vi "Do.vi"(8 "error in (no error)":errorcluster, 10 "Actor in":refnum<class "Actor.lvclass">, 11 "PID Actor Msg":refnum<class "PID Actor Msg.lvclass">) -> (0 "error out":errorcluster, 2 "Actor out":refnum<class "Actor.lvclass">)   [LabVIEW 2024, in "PID Actor.lvlib" / "PID Actor Msg.lvclass"]
doc: "(<B>Filename</B>: Actor Framework.lvlib:Message.lvclass:Do.vi)\n\nDefines what a message does when it is received by an actor. Generally, a message instructs an actor to invoke one of its methods. By default, this method does nothing. A child class must override it to define behavior. Create a child class by using the Actor Framework Message Maker dialog box."
uses:
  PID Actor Msg.lvclass
  <vilib>/ActorFramework/Actor/Actor.lvclass
  Actor/PID.lvclass
  C:/Program Files (x86)/National Instruments/LabVIEW 2024/vi.lib/ActorFramework/Actor/Actor.lvclass
  PID Actor Msg.lvclass/PID Actor Msg.ctl
  <vilib>/ActorFramework/Message/Message.lvclass
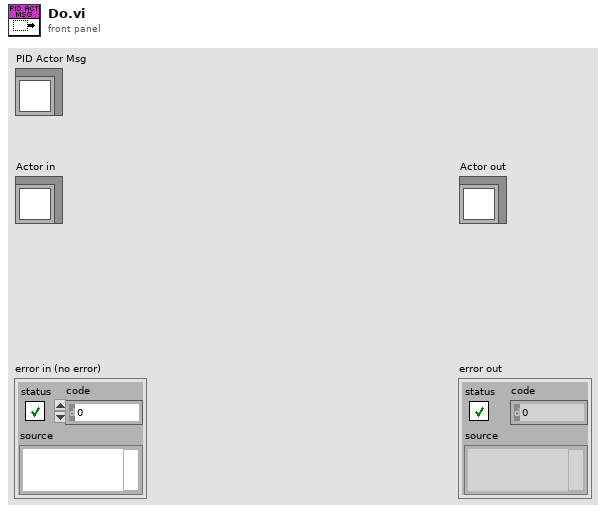
[diagram p1: front panel]
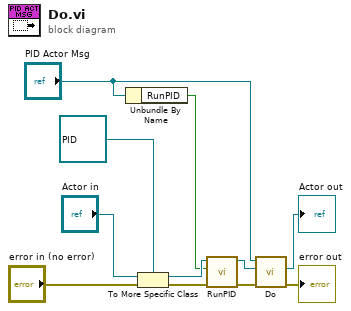
[diagram p0: block diagram]
diagram:
  n1 = Unbundle By Name("PID Actor Msg") -> ("RunPID"=w4:bool)
  n2 = To More Specific Class(target class=refnum<class "PID.lvclass"> refnum ("PID Actor.lvlib:PID.lvclass"), reference="Actor in", error in="error in (no error)") -> (specific class reference=w6:refnum<class "PID.lvclass">, error out=w5:errorcluster)
  n3 = call "RunPID.vi"("error in (no error)"=w5, "Run"=w4, "PID in"=w6) -> ("error out"=w1:errorcluster, "PID out"=w2:refnum<class "PID.lvclass">)  [unwired: 7 in]
  n4 = call-parent "Do.vi"("error in (no error)"=w1, "Actor in"=w2, "Message"="PID Actor Msg") -> ("error out"=→"error out":errorcluster, "Actor out"=→"Actor out":refnum<class "Actor.lvclass">)  [unwired: 7 in]
